vi "Resize Array of Strings.vi"(8 "Error In":errorcluster, 9 "dimension size":i32=10, 10 "Array":string[](array[string])) -> (0 "Error Out":errorcluster, 2 "output array":string[](array[string]))   [LabVIEW 2016, in "TL27.lvlib"]
uses:
  Projects/TL27.lvlib
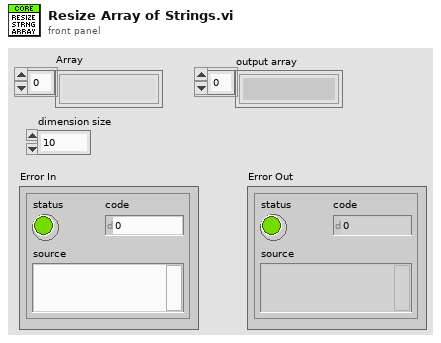
[diagram p1: front panel]
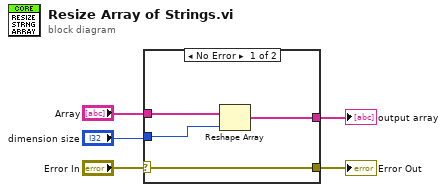
[diagram p0: block diagram]
diagram:
  n1 = case shown="No Error" "Error In" {
    selector: "Error In" -> [w6 w11]
    tunnel: "Array" -> [w9 w10]
    tunnel: "dimension size" -> [w8 _]
    tunnel: [w7 w10] -> w3
    tunnel: [w6 w11] -> w1
    frame No Error {
      n2 = Reshape Array(w9, w8) -> (w7:string[])
    }
    frame Error {
    }
  }
  "output array" <- w3
  "Error Out" <- w1
